vi "Delete Group.vi"(8 "error in (no error)":errorcluster, 11 "Group":string) -> (0 "error out":errorcluster)   [LabVIEW 2010, in "Current Value Table.lvlib"]
doc: "Deletes a group by name. This does not delete the associated tags. Attempting to read or write this group from a node that has not yet been called will throw an error. Attempting to read or write this group from a node which has already been called has undefined behavior as the tag lookup has already been performed."
uses:
  Current Value Table.lvlib
  FGVs/Group Memory Methods.ctl
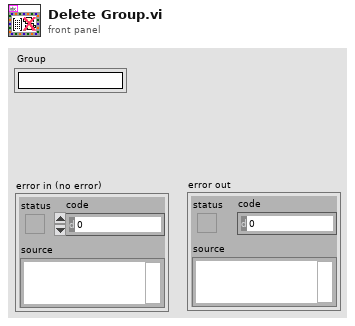
[diagram p1: front panel]
types:
  T1 = typedef "Current Value Table.lvlib/Group Memory Methods.ctl" = enum16{"Clear", "Read Indices in Group", "List Groups", "List Tags by Type", "List Tags", "Delete Group", "Check Group Existence", "Create Group"}
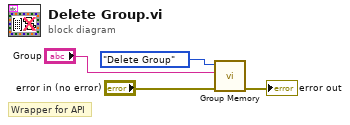
[diagram p0: block diagram]
diagram:
  # "Wrapper for API"
  n1 = call "Group Memory.vi"("error in (no error)"="error in (no error)", "Group"="Group", "Method"=Group_Memory_Methods."Delete Group") -> ("error out"=→"error out":errorcluster)  [unwired: 5 in, 3 out]
